vi "Active Command.vi"() -> ()   [LabVIEW 2017]
uses:
  AutonBuilder/Typedef/Single Sequence.ctl
  AutonBuilder/Typedef/Sequence Command.ctl
  AutonBuilder/Typedef/Plate Arrangement.ctl
panel:
  in  "Auton Sequence":T1[](array[typedef])
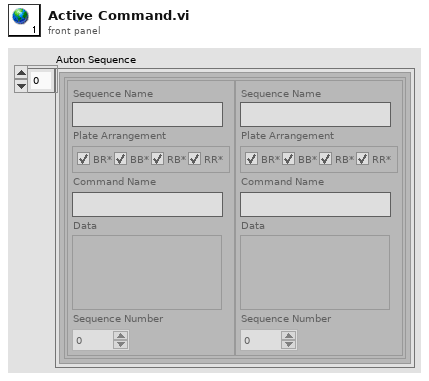
[diagram p1: front panel]
types:
  T1 = typedef "Single Sequence.ctl" = cluster{"Sequence Array":T2[]}
  T2 = typedef "Sequence Command.ctl" = cluster{"Sequence Name":string, "Plate Arrangement":T3, "Command Name":string, "Data":variant, "Sequence Number":u32}
  T3 = typedef "Plate Arrangement.ctl" = cluster{"BR*":bool, "BB*":bool, "RB*":bool, "RR*":bool}
diagram:
